vi "StartSplashScreen.vi"(8 "error in (no error)":errorcluster) -> (0 "error out":errorcluster)   [LabVIEW 2013]
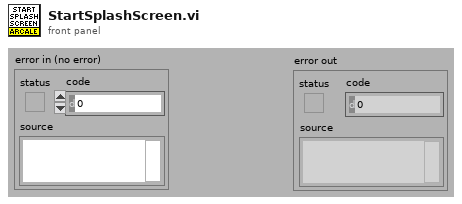
[diagram p1: front panel]
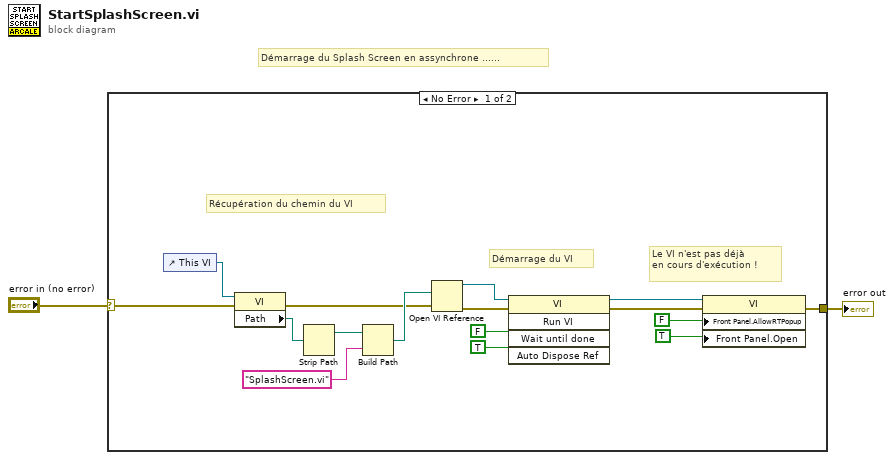
[diagram p0: block diagram]
diagram:
  # "Démarrage du Splash Screen en assynchrone ......"
  n1 = case shown="No Error" "error in (no error)" {
    selector: "error in (no error)" -> [w16 w19]
    tunnel: [w18 w19] -> w2
    frame No Error {
      # "Le VI n'est pas déjà\nen cours d'exécution !"
      # "Démarrage du VI"
      # "Récupération du chemin du VI"
      n2 = control-ref of="This VI"() -> (w17:refnum<vi>)
      n3 = property class="VI"(reference=w17, error in=w16) -> (error out=w10:errorcluster, "Path"=w15:path)  [unwired: 1 out]
      n4 = Strip Path(path=w15) -> (stripped path=w14:path)  [unwired: 1 out]
      n5 = Build Path(base path=w14, name or relative path="SplashScreen.vi") -> (appended path=w11:path)
      n6 = Open VI Reference(vi path=w11, error in (no error)=w10) -> (vi reference=w9:refnum<vi>, error out=w12:errorcluster)  [unwired: 4 in]
      n7 = invoke class="VI" method="Run VI"(reference=w9, error in=w12, "Wait until done"=FALSE ("Wait Until Done"), "Auto Dispose Ref"=TRUE ("Auto Dispose Reference")) -> (reference out=w4:refnum<vi>, error out=w3:errorcluster)  [unwired: 1 in, 3 out]
      n8 = property class="VI"(reference=w4, error in=w3, "Front Panel.AllowRTPopup"=FALSE ("Front Panel Window:Allow Runtime PopUp"), "Front Panel.Open"=TRUE ("Front Panel Window:Open")) -> (error out=w18:errorcluster)  [unwired: 1 out]
    }
    frame Error {
    }
  }
  "error out" <- w2
